vi "SR430_bin_width_2_us.vi"(2 "bin width":i32, 5 "error in (no error)":errorcluster) -> (16 "binWidth [us]":dbl format="%.3f", 17 "InRange?":bool, 19 "error out":errorcluster)   [LabVIEW 2009, in "SR430Driver.lvlib"]
doc: "converts the bin width in the format used by the unit into mircoseconds.\n\nVI Tree for the SR430 Multi-Channel Scaler from Staford Research Systems.\n\nHistory: 24-APR-2002, Dietrich Beck\n\nCopyright (C)\nGesellschaft für Schwerionenforschung, GSI\nPlanckstr. 1\n64291 Darmstadt\nGermany\n\nContact: D.Beck@gsi.de \n\nThis program is free software; you can redistribute it and/or modify it under the terms of the \nGNU General Public License as published by the Free Software Foundation; either version 2 of the license, or (at your option) any later version.\n\nThis program is distributed in the hope that it will be useful, but WITHOUT ANY WARRANTY; without even the implied warranty of MERCHANTABILITY or FITNESS FOR A PARTICULAR PURPOSE. See the GNU General License for more details (http://www.gnu.org).\n\nGesellschaft für Schwerionenforschung, GSI\nPlanckstr. 1, 64291 Darmstadt, Germany\nFor all questions and ideas contact: M.Richter@gsi.de, K.Poppensieker, H.Brand@gsi.de or D.Beck@gsi.de.\nLast update: 11-APR-2002"
uses:
  SR430Driver.lvlib
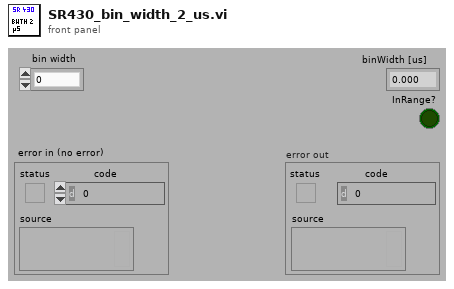
[diagram p1: front panel]
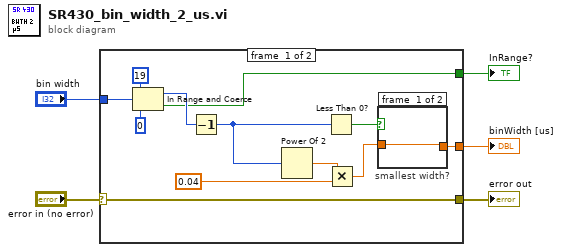
[diagram p0: block diagram]
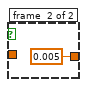
[diagram p2: hidden frame]
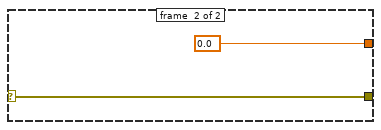
[diagram p3: hidden frame]
diagram:
  n1 = case shown="No Error" "error in (no error)" {
    selector: "error in (no error)" -> [w11 w21]
    tunnel: [w13 0.0 ("Ist-Gate [us]")] -> w5
    tunnel: "bin width" -> [w10 _]
    tunnel: [w11 w21] -> w2
    tunnel: [w6 _] -> w1
    frame #0 {
      n2 = In Range and Coerce(upper limit=19, x=w10, lower limit=0) -> (coerced(x)=w7:i32, In Range?=w6:bool)
      n3 = Decrement(x=w7) -> (x-1=w12:i32)
      n4 = Power Of 2(x=w12) -> (2^x=w17:dbl)
      n5 = Less Than 0?(x=w12) -> (x < 0?=w15:bool)
      n6 = Multiply(x=w17, y=0.04) -> (x*y=w16:dbl)
      n7 = case "smallest width?" shown="True" w15 {
        tunnel: [w18 0.005 ("Ist-Gate [us]")] -> w13
        tunnel: w16 -> [w18 _]
        frame #0 {
        }
        frame #1 {
        }
      }
    }
    frame #1 {
    }
  }
  "error out" <- w2
  "binWidth [us]" <- w5
  "InRange?" <- w1
